vi "Top_Level_DDE.vi"() -> ()   [LabVIEW 2013]
uses:
  DE/Controls/Instance_Type.ctl
  DE/Controls/States_DDE.ctl
  OSSP_Problem.lvclass
panel:
  in  "Instance Type":T1
  out "error out":errorcluster
  in  "error in (no error)":errorcluster
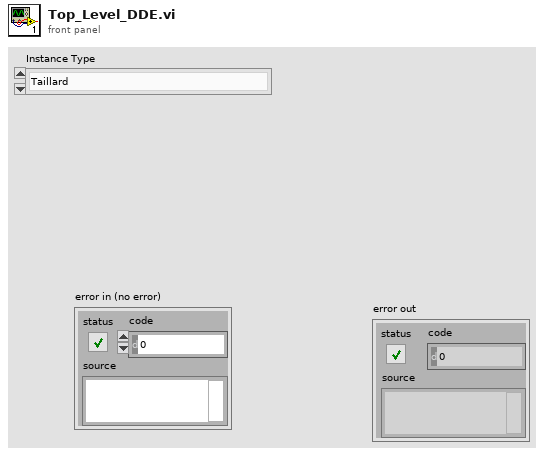
[diagram p1: front panel]
types:
  T1 = typedef "Instance_Type.ctl" = enum16{"Taillard", "Brucker", "Gueret-Prins"}
  T2 = typedef "States_DDE.ctl" = enum16{"Read Problem", "Stop"}
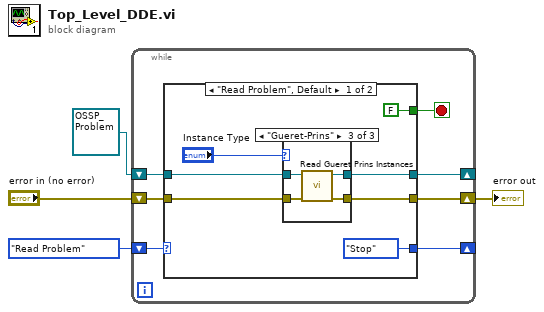
[diagram p0: block diagram]
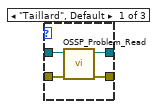
[diagram p2: hidden frame]
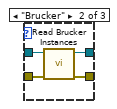
[diagram p3: hidden frame]
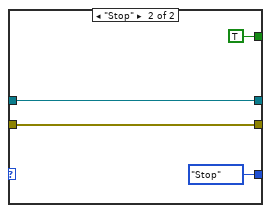
[diagram p4: hidden frame]
diagram:
  n1 = while {
    shift-right: [w9] -> _
    shift-left: States_DDE."Read Problem" -> [w11]
    shift-right: [w5] -> _
    shift-left: refnum<class "OSSP_Problem.lvclass"> refnum ("OSSP_Problem.lvclass") -> [w8]
    shift-right: [w6] -> w1
    shift-left: "error in (no error)" -> [w7]
    stop <- w10 stop-if-true
    n2 = case shown="\"Read Problem\", Default" w11 {
      tunnel: [FALSE TRUE] -> w10
      tunnel: [States_DDE."Stop" States_DDE."Stop"] -> w9
      tunnel: w8 -> [w17 w31]
      tunnel: w7 -> [w16 w32]
      tunnel: [w15 w32] -> w6
      tunnel: [w13 w31] -> w5
      frame "Read Problem", Default {
        n3 = case shown="\"Gueret-Prins\"" "Instance Type" {
          tunnel: w17 -> [w22 w26 w30]
          tunnel: w16 -> [w21 w24 w28]
          tunnel: [w20 w23 w27] -> w15
          tunnel: [w19 w25 w29] -> w13
          frame "Taillard", Default {
            n4 = call "OSSP_Problem_Read.vi"("error in (no error)"=w21, "OSSP_Problem.lvclass In"=w22) -> ("error out"=w20:errorcluster, "OSSP_Problem.lvclass Out"=w19:refnum<class "OSSP_Problem.lvclass">)  [unwired: 6 in, 2 out]
          }
          frame "Brucker" {
            n5 = call "Read Brucker Instances.vi"("error in (no error)"=w24, "OSSP_Problem in"=w26) -> ("error out"=w23:errorcluster, "OSSP_Problem out"=w25:refnum<class "OSSP_Problem.lvclass">)  [unwired: 7 in, 1 out]
          }
          frame "Gueret-Prins" {
            n6 = call "Read Gueret Prins Instances.vi"("error in (no error)"=w28, "OSSP_Problem in"=w30) -> ("error out"=w27:errorcluster, "OSSP_Problem out"=w29:refnum<class "OSSP_Problem.lvclass">)  [unwired: 7 in, 1 out]
          }
        }
      }
      frame "Stop" {
      }
    }
  }
  "error out" <- w1
